vi "Stager.vi"(6 "Files Generated by Build":path[](array[path]), 8 "error in (no error)":errorcluster, 9 "Product":string, 10 "Vendor":string, 11 "Destination Path":path) -> (0 "error out":errorcluster, 3 "Staged Path":path)   [LabVIEW 2016]
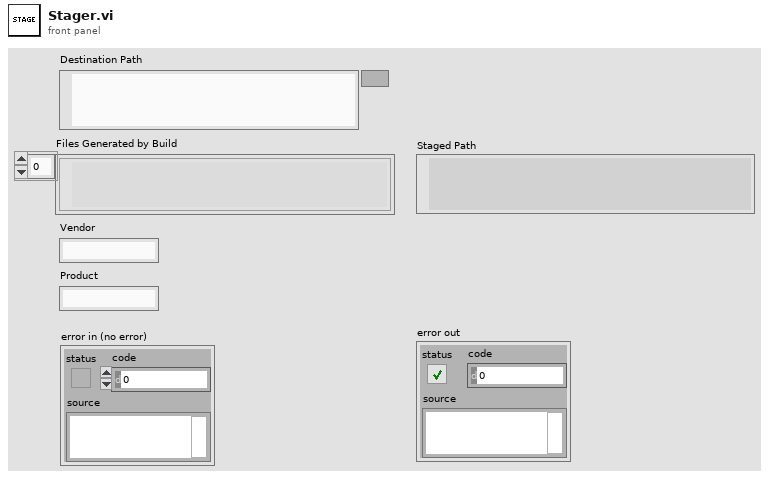
[diagram p1: front panel]
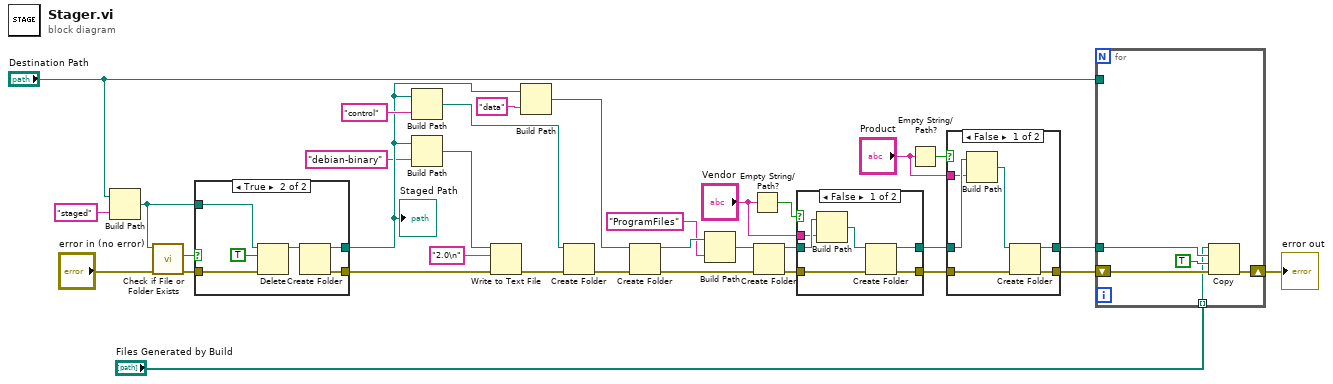
[diagram p0: block diagram]
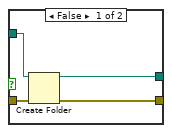
[diagram p4: hidden frame]
diagram:
  n1 = Build Path(base path="Destination Path", name or relative path="staged") -> (appended path=w31:path)
  n2 = call <vilib>:"Check if File or Folder Exists.vi"("error in (no error)"="error in (no error)", "path"=w31) -> ("error out"=w29:errorcluster, "file or folder exists?"=w32:bool)  [unwired: 7 in, 1 out]
  n3 = case shown="True" w32 {
    tunnel: w31 -> [w37 w43]
    tunnel: [w36 w40] -> w8
    tunnel: w29 -> [w34 w39]
    tunnel: [w35 w38] -> w4
    frame False {
      n4 = Create Folder(path (use dialog)=w37, error in=w34) -> (created path=w36:path, error out=w35:errorcluster)  [unwired: 1 in, 1 out]
    }
    frame True {
      n5 = Delete(path (use dialog)=w43, entire hierarchy (F)=TRUE, error in=w39) -> (deleted path=w41:path)  [unwired: 2 in, 2 out]
      n6 = Create Folder(path (use dialog)=w41) -> (created path=w40:path, error out=w38:errorcluster)  [unwired: 2 in, 1 out]
    }
  }
  "Staged Path" <- w8
  n7 = Build Path(base path=w8, name or relative path="control") -> (appended path=w26:path)
  n8 = Build Path(base path=w8, name or relative path="debian-binary") -> (appended path=w6:path)
  n9 = Write to Text File(file (use dialog)=w6, text="2.0\n", error in=w4) -> (error out=w3:errorcluster)  [unwired: 1 in, 2 out]
  n10 = Build Path(base path=w8, name or relative path="data") -> (appended path=w27:path)
  n11 = Create Folder(path (use dialog)=w26, error in=w3) -> (error out=w25:errorcluster)  [unwired: 1 in, 2 out]
  n12 = Create Folder(path (use dialog)=w27, error in=w25) -> (created path=w24:path, error out=w23:errorcluster)  [unwired: 1 in, 1 out]
  n13 = Build Path(base path=w24, name or relative path="ProgramFiles") -> (appended path=w22:path)
  n14 = Empty String/Path?(string/path="Vendor") -> (empty?=w17:bool)
  n15 = Create Folder(path (use dialog)=w22, error in=w23) -> (created path=w20:path, error out=w12:errorcluster)  [unwired: 1 in, 1 out]
  n16 = case shown="False" w17 {
    tunnel: w20 -> [w48 w51]
    tunnel: [w47 w51] -> w19
    tunnel: "Vendor" -> [w46 _]
    tunnel: w12 -> [w45 w50]
    tunnel: [w44 w50] -> w11
    frame False {
      n17 = Build Path(base path=w48, name or relative path=w46) -> (appended path=w49:path)
      n18 = Create Folder(path (use dialog)=w49, error in=w45) -> (created path=w47:path, error out=w44:errorcluster)  [unwired: 1 in, 1 out]
    }
    frame True {
    }
  }
  n19 = Empty String/Path?(string/path="Product") -> (empty?=w15:bool)
  n20 = case shown="False" w15 {
    tunnel: w19 -> [w56 w59]
    tunnel: "Product" -> [w55 _]
    tunnel: [w54 w59] -> w14
    tunnel: w11 -> [w53 w58]
    tunnel: [w52 w58] -> w10
    frame False {
      n21 = Build Path(base path=w56, name or relative path=w55) -> (appended path=w57:path)
      n22 = Create Folder(path (use dialog)=w57, error in=w53) -> (created path=w54:path, error out=w52:errorcluster)  [unwired: 1 in, 1 out]
    }
    frame True {
    }
  }
  n23 = for {
    tunnel: w14 -> [w63]
    tunnel: "Destination Path" -> [_]
    shift-right: [w61] -> w9
    shift-left: w10 -> [w62]
    tunnel: "Files Generated by Build" -> [w60] mode=indexing
    n24 = Copy(8:w62, 9:TRUE ("overwrite (F)"), 10:w63, 11:w60) -> (0:w61:errorcluster)  [unwired: 1 in, 2 out]
  }
  "error out" <- w9
